vi "isMapRun.vi"() -> ()   [LabVIEW 2024]
panel:
  in  "Is Map running":bool
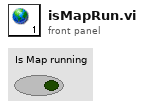
[diagram p1: front panel]
diagram:
